vi "Get Region.vi"(8 "error in (no error)":errorcluster, 11 "Camera in":refnum<class "Camera.lvclass">) -> (0 "error out":errorcluster, 1 "Region Size":T1, 2 "Region Offset":T2, 3 "Camera":refnum<class "Camera.lvclass">)   [LabVIEW 2020, in "Camera.lvclass"]
uses:
  Camera.lvclass
  Image Offset.ctl
  Buffer/Image Size.ctl
  Camera.lvclass/Camera.ctl
  Check Not Disconnected.vi
  <vilib>/Utility/error.llb/Error Cluster From Error Code.vi
  Buffer/Buffer.lvclass
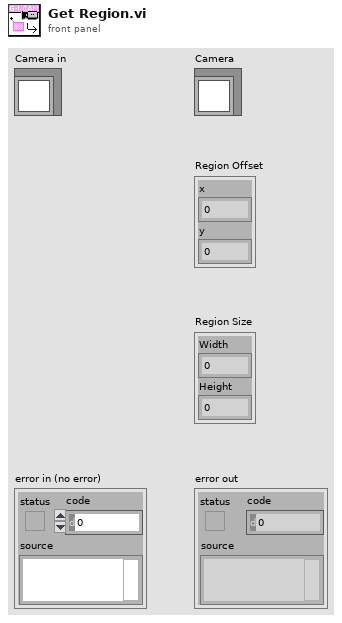
[diagram p1: front panel]
types:
  T1 = typedef "Buffer.lvclass/Image Size.ctl" = cluster{"Width":u16, "Height":u16}
  T2 = typedef "Camera.lvclass/Image Offset.ctl" = cluster{"x":i32, "y":i32}
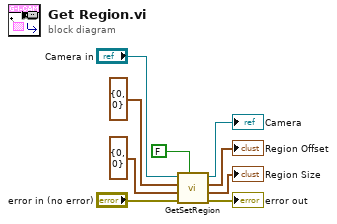
[diagram p0: block diagram]
diagram:
  n1 = call "GetSetRegion.vi"("Set"=FALSE, "error in (no error)"="error in (no error)", "Image Size"=T1 {"Width"=0, "Height"=0}, "Image Offset"=T2 {"x"=0, "y"=0}, "Camera in"="Camera in") -> ("error out"=→"error out":errorcluster, "Image Size"=→"Region Size":T1, "Image Offset"=→"Region Offset":T2, "Camera"=→"Camera":refnum<class "Camera.lvclass">)  [unwired: 3 in]
